vi "AddItem.vi"(6 "Veg":bool, 7 "Price":i32, 8 "Error In":errorcluster, 9 "Description":string, 10 "Name":string, 11 "reference in":refnum<class "BreakfastMenu.lvclass">) -> (0 "Error Out":errorcluster, 3 "reference out":refnum<class "BreakfastMenu.lvclass">)   [LabVIEW 2020, in "BreakfastMenu.lvclass"]
uses:
  BreakfastMenu.lvclass
  Menu_class/Menu.lvclass
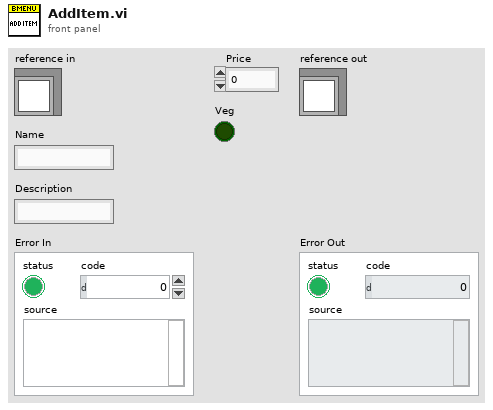
[diagram p1: front panel]
types:
  T1 = typedef "BreakfastMenu.lvclass/ObjectAttributes.ctl" = cluster{"_items":refnum<class "Menu.lvclass">[], "Items":refnum<class "IEnumerable.lvclass">}
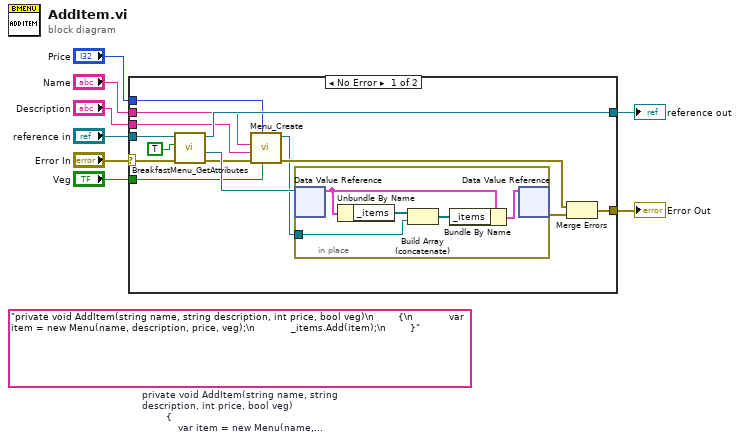
[diagram p0: block diagram]
diagram:
  (unwired) "private void AddItem(string name, string description, int price, bool veg)\n        {\n            var item = new Menu(name, description, price, veg);\n            _items.Add(item);\n        }"  # private void AddItem(string name, string description, int price, bool veg)         {             var item = new Menu(name, description, price, veg);             _items.Add(item);         }
  n1 = case shown="No Error" "Error In" {
    selector: "Error In" -> [w21 w29]
    tunnel: [w18 w29] -> w7
    tunnel: [w19 w28] -> w5
    tunnel: "reference in" -> [w22 w28]
    tunnel: "Price" -> [w15 _]
    tunnel: "Name" -> [w14 _]
    tunnel: "Description" -> [w13 _]
    tunnel: "Veg" -> [w12 _]
    frame No Error {
      n2 = call "BreakfastMenu_GetAttributes.vi"("error in (no error)"=w21, "OnlyGetDvrReference(False)"=TRUE, "reference in"=w22) -> ("error out"=w11:errorcluster, "DataRef"=w17:refnum<data-value>, "reference out"=w19:refnum<class "BreakfastMenu.lvclass">)  [unwired: 5 in, 1 out]
      n3 = call "Menu_Create.vi"("Vegetarian"=w12, "Price"=w15, "Error In"=w11, "Description"=w13, "Name"=w14) -> ("Error Out"=w10:errorcluster, "reference out"=w9:refnum<class "Menu.lvclass">)  [unwired: 5 in]
      n4 = in-place {
        in-place-border: w9 -> [w24]
        n5 = in-place-dvr #1(w17) -> (w26:T1)  [unwired: 1 out]
        n6 = Unbundle By Name(w26) -> ("_items"=w25:refnum<class "Menu.lvclass">[])
        n7 = Build Array (concatenate)(w25, w24) -> (w23:refnum<class "Menu.lvclass">[])
        n8 = Bundle By Name(cluster=w26, "_items"=w23) -> (w27:T1)
        n9 = in-place-dvr #1(w27) -> (w20:errorcluster)  [unwired: 1 out]
      }
      n10 = Merge Errors(w10, w20) -> (w18:errorcluster)
    }
    frame Error {
    }
  }
  "Error Out" <- w7
  "reference out" <- w5
